vi "Limelight HatchPanel.vi"() -> ()   [LabVIEW 2018]
uses:
  <vilib>/Rock Robotics/Network Tables/NT Read Number.vi
panel:
  in  "allowed error":dbl
  in  "kpDist":dbl
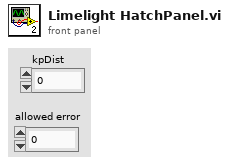
[diagram p1: front panel]
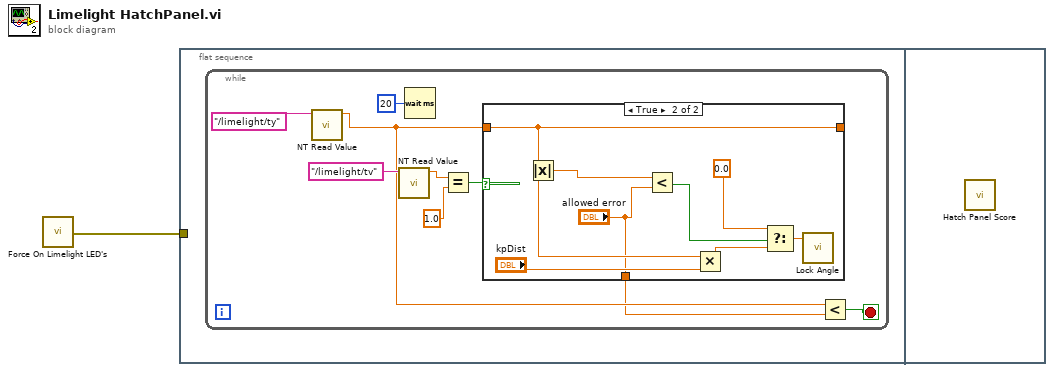
[diagram p0: block diagram]
diagram:
  n1 = call "Force On Limelight LED's.vi"() -> ("error out"=w1:errorcluster)  [unwired: 10 in]
  n2 = flat-sequence {
    tunnel: w1 -> [_]
    frame #0 {
      n3 = while {
        stop <- w5 stop-if-true
        n4 = call-poly <vilib>:"NT Read Value.vi"("Name"="/limelight/ty") -> ("Numeric"=w4:dbl)  [unwired: 9 in, 1 out]
        n5 = call-poly <vilib>:"NT Read Value.vi"("Name"="/limelight/tv") -> ("Numeric"=w9:dbl)  [unwired: 9 in, 1 out]
        n6 = Wait (ms)(milliseconds to wait=u32 20) -> ()  [unwired: 1 out]
        n7 = Equal?(x=w9, y=1.0) -> (x = y?=w7:bool)
        n8 = case shown="True" w7 {
          tunnel: [w11 w18] -> _
          tunnel: w4 -> [w11 w18]
          tunnel: [_ "allowed error"] -> w3
          frame False {
          }
          frame True {
            n9 = Absolute Value(x=w18) -> (abs(x)=w17:dbl)
            n10 = Less?(x=w17, y="allowed error") -> (x < y?=w14:bool)
            n11 = Multiply(x=w18, y="kpDist") -> (x*y=w15:dbl)
            n12 = Select(t=0.0, s=w14, f=w15) -> (s? t:f=w13:dbl)
            n13 = call "Lock Angle.vi"("Setpoint"=w13) -> ()  [unwired: 11 in]
          }
        }
        n14 = Less?(x=w4, y=w3) -> (x < y?=w5:bool)
      }
    }
    frame #1 {
      n15 = call "Hatch Panel Score.vi"() -> ()  [unwired: 11 in, 1 out]
    }
  }
